vi "Close Module.vi"(8 "error in":errorcluster, 11 "Module Admin in":refnum<class "Delacor_lib_QMH_Module Admin.lvclass">) -> (0 "error out":errorcluster, 1 "External Launch":bool, 3 "Module Admin out":refnum<class "Delacor_lib_QMH_Module Admin.lvclass">)   [LabVIEW 2020, in "Logger.lvlib"]
doc: "Destroy the Broadcast Events and Request Events. Reset flags stored in Module Admin class.\n_____\nBased on DQMH Project Template 4.0.0.47.\n_____\nBased on DQMH Project Template 7.0.1.1316."
uses:
  Logger.lvlib
  <vilib>/Delacor/Delacor QMH/Libraries/Module Admin_class/Delacor_lib_QMH_Module Admin.lvclass
  <vilib>/Delacor/Delacor QMH/Libraries/Module Admin_class/Delacor_lib_QMH_Module Admin.lvclass/Delacor_lib_QMH_Module Admin.ctl
  <vilib>/Delacor/Delacor QMH/Libraries/Module Admin_class/Delacor_lib_QMH_Get External Launch.vi
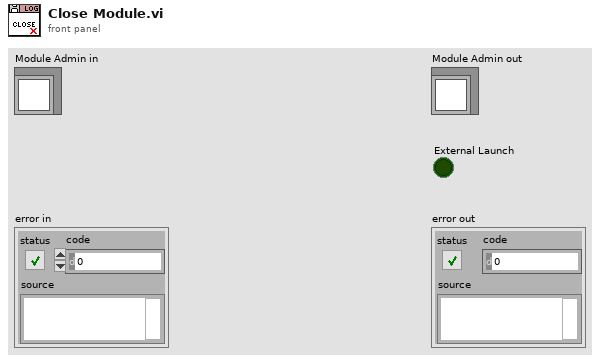
[diagram p1: front panel]
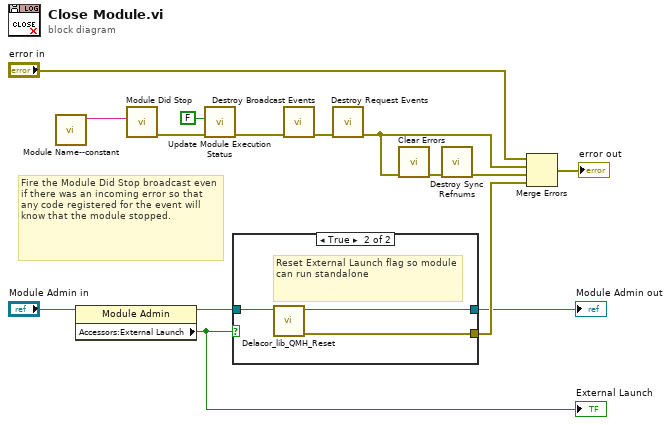
[diagram p0: block diagram]
diagram:
  # "Fire the Module Did Stop broadcast even if there was an incoming error so that any code registered for the event will know that the module stopped."
  n1 = call "Module Name--constant.vi"() -> ("Module Name"=w8:string)  [unwired: 11 in]
  n2 = property on="Property Node" class="Module Admin"(reference="Module Admin in") -> (reference out=w13:refnum<class "Delacor_lib_QMH_Module Admin.lvclass">, "Accessors:External Launch"=w10:bool)  [unwired: 1 in, 1 out]
  "External Launch" <- w10
  n3 = call "Module Did Stop.vi"("Origin"=w8) -> ("error out"=w7:errorcluster)  [unwired: 10 in]
  n4 = call "Update Module Execution Status.vi"("error in"=w7, "Running?"=FALSE) -> ("error out"=w2:errorcluster)  [unwired: 9 in]
  n5 = case shown="True" w10 {
    tunnel: w13 -> [w16 w19]
    tunnel: [w16 w18] -> w11
    tunnel: [_ w17] -> w15
    frame False {
    }
    frame True {
      # "Reset External Launch flag so module can run standalone"
      n6 = call-dynamic "Delacor_lib_QMH_Reset.vi"("Mod Admin in"=w19) -> ("error out"=w17:errorcluster, "Mod Admin out"=w18:refnum<class "Delacor_lib_QMH_Module Admin.lvclass">)  [unwired: 9 in]
    }
  }
  "Module Admin out" <- w11
  n7 = call "Destroy Broadcast Events.vi"("error in"=w2) -> ("error out"=w9:errorcluster)  [unwired: 10 in]
  n8 = call "Destroy Request Events.vi"("error in"=w9) -> ("error out"=w14:errorcluster)  [unwired: 10 in]
  n9 = call <vilib>:"Clear Errors.vi"("error in (no error)"=w14) -> ("error out"=w4:errorcluster)  [unwired: 5 in, 1 out]
  n10 = call "Destroy Sync Refnums.vi"("error in"=w4) -> ("error out"=w6:errorcluster)  [unwired: 10 in]
  n11 = Merge Errors("error in", w14, w6, w15) -> (→"error out":errorcluster)
